vi "SaveParamsToGlobalExp.vi"(8 "error in":errorcluster, 11 "FlattendJSon in":string) -> (0 "error out":errorcluster, 2 "steps":i32, 3 "FlattendJSon out":string)   [LabVIEW 2019]
uses:
  controls/GlobalExp.vi
  Global.lvlib
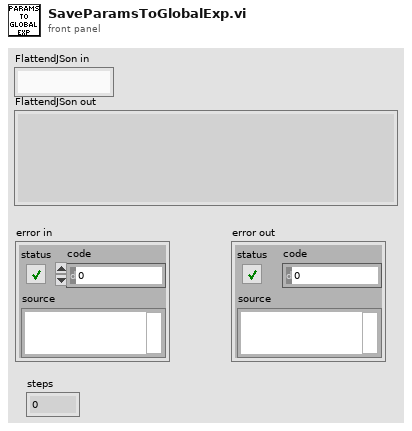
[diagram p1: front panel]
types:
  T1 = typedef "MasterExpControl.ctl" = cluster{"Main Steps":dbl, "Main Runs":dbl, "ExpStatus":enum16{"Innit", "Stop", "Idle", "MainRunning", "AuxRunning"}, "Main Current Step":dbl, "ExpNum":dbl, "NewData":bool, "date":string, "command":string, "Stop":bool, "Pause":bool, "Mathematica":string, "Main/Meta":bool, "UpdateMath":bool, "Camera":bool, "MetaExpOver":bool, "NextMetaExp":bool}
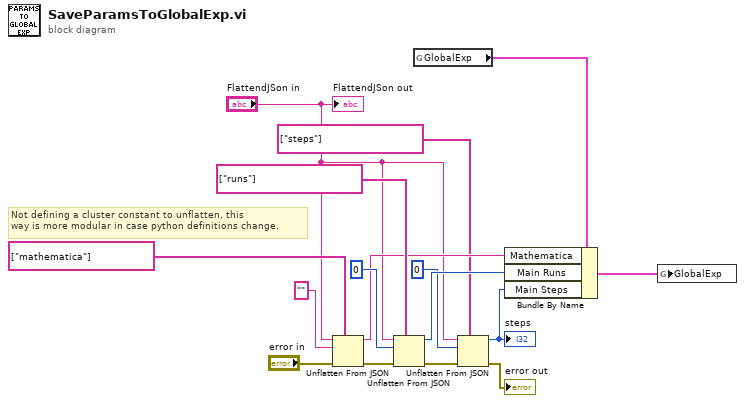
[diagram p0: block diagram]
diagram:
  # "Not defining a cluster constant to unflatten, this \nway is more modular in case python definitions change."
  n1 = Unflatten From JSON(path=string[] ["mathematica"], JSON string="FlattendJSon in", type and defaults="", error in (no error)="error in") -> (value=w10:string, error out=w3:errorcluster)  [unwired: 3 in]
  n2 = Unflatten From JSON(path=string[] ["runs"], JSON string="FlattendJSon in", type and defaults=0, error in (no error)=w3) -> (value=w9:i32, error out=w2:errorcluster)  [unwired: 3 in]
  n3 = global read "GlobalExp.vi" "GlobalExp"() -> (w11:T1)
  n4 = Unflatten From JSON(path=string[] ["steps"], JSON string="FlattendJSon in", type and defaults=0, error in (no error)=w2) -> (value=w6:i32, error out=→"error out":errorcluster)  [unwired: 3 in]
  "steps" <- w6
  n5 = Bundle By Name(cluster=w11, "Mathematica"=w10, "Main Runs"=w9, "Main Steps"=w6) -> (w12:T1)
  n6 = global write "GlobalExp.vi" "GlobalExp"(w12) -> ()
  "FlattendJSon out" <- "FlattendJSon in"
